vi "XTicks2000.vi"   [LabVIEW 2013]
uses:
  <vilib>/Heliosphere Research LLC/Advanced Plotting Toolkit/Advanced Plotting Toolkit.lvlib
types:
  T1 = typedef "Advanced Plotting Toolkit.lvlib/PlotID.ctl" = i32
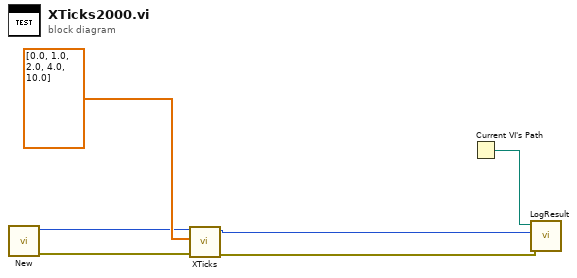
[diagram p0: block diagram]
diagram:
  n1 = call <vilib>:"New.vi"() -> ("error out"=w3:errorcluster, "Plot ID"=w4:T1)  [unwired: 10 in]
  n2 = call <vilib>:"XTicks.vi"("error in (no error)"=w3, "Tick Locations"=dbl[] [0.0, 1.0, 2.0, 4.0, 10.0], "Plot ID"=w4) -> ("error out"=w2:errorcluster, "Plot ID Out"=w1:T1)  [unwired: 7 in]
  n3 = Current VI's Path() -> (path=w6:path)
  n4 = call "LogResult.vi"("Test Result"=w2, "Test Artifact"=w1, "VI Path"=w6) -> ()  [unwired: 9 in]
